vi "Part 2.vi"(11 "Input":string) -> (3 "Output":i64)   [LabVIEW 2021]
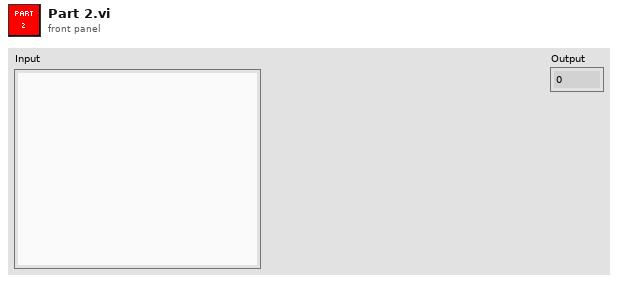
[diagram p1: front panel]
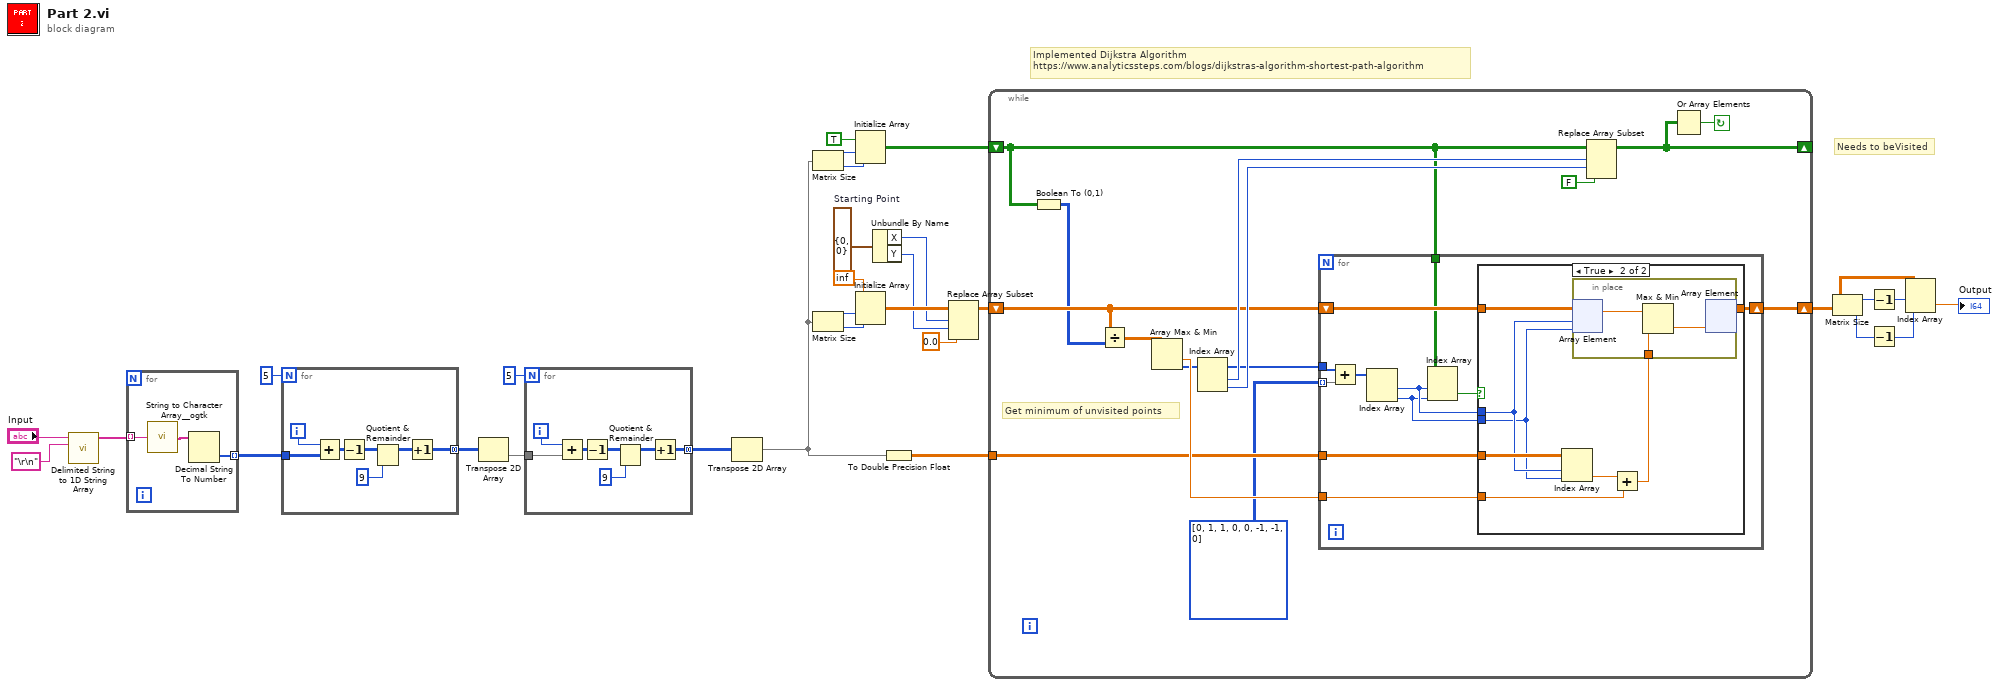
[diagram p0: block diagram]
diagram:
  w18 = cluster{"X":i32, "Y":i32} {"X"=0, "Y"=0}  # Starting Point
  # "Implemented Dijkstra Algorithm\nhttps://www.analyticssteps.com/blogs/dijkstras-algorithm-shortest-path-algorithm"
  # "Needs to beVisited"
  n1 = call <vilib>:"Delimited String to 1D String Array.vi"("delimiter"="\r\n", "delimited string"="Input") -> ("string array"=w29:string[])  [unwired: 9 in]
  n2 = for {
    tunnel: w29 -> [w33] mode=indexing
    tunnel: [w31] -> w9 mode=indexing
    n3 = call <userlib>:"String to Character Array__ogtk.vi"("Input String"=w33) -> ("Character Array"=w32:string[])
    n4 = Decimal String To Number(string=w32) -> (number=w31:i32[])  [unwired: 2 in, 1 out]
  }
  n5 = for {
    N: 5 -> [_]
    tunnel: w9 -> [w39]
    tunnel: [w37] -> w7 mode=concatenating
    i -> [w40]
    n6 = Add(x=w40, y=w39) -> (x+y=w38:i32[][])
    n7 = Decrement(x=w38) -> (x-1=w36:i32[][])
    n8 = Quotient & Remainder(x=w36, y=9) -> (x-y*floor(x/y)=w35:i32[][])  [unwired: 1 out]
    n9 = Increment(x=w35) -> (x+1=w37:i32[][])
  }
  n10 = Transpose 2D Array(2D array=w7) -> (transposed array=w5:i32[][])
  n11 = for {
    N: 5 -> [_]
    tunnel: w5 -> [w46]
    tunnel: [w41] -> w4 mode=concatenating
    i -> [w47]
    n12 = Add(x=w47, y=w46) -> (x+y=w42:i32[][])
    n13 = Decrement(x=w42) -> (x-1=w45:i32[][])
    n14 = Quotient & Remainder(x=w45, y=9) -> (x-y*floor(x/y)=w44:i32[][])  [unwired: 1 out]
    n15 = Increment(x=w44) -> (x+1=w41:i32[][])
  }
  n16 = Transpose 2D Array(2D array=w4) -> (transposed array=w2:i32[][])
  n17 = Matrix Size(0:w2) -> (1:w28:i32, 2:w27:i32)
  n18 = Matrix Size(0:w2) -> (1:w21:i32, 2:w22:i32)
  n19 = Initialize Array(TRUE, w28, w27) -> (w25:bool[][])
  n20 = Initialize Array(inf, w21, w22) -> (w23:dbl[][])
  n21 = Unbundle By Name(w18) -> ("X"=w16:i32, "Y"=w17:i32)
  n22 = To Double Precision Float(number=w2) -> (double precision float=w1:dbl[][])
  n23 = Replace Array Subset(array=w23, new element=0.0, index (row)=w16, index (col)=w17) -> (w19:dbl[][])
  n24 = while {
    shift-right: [w53] -> _
    shift-left: w25 -> [w48]
    shift-right: [w59] -> w10
    shift-left: w19 -> [w55]
    tunnel: w1 -> [w52]
    stop <- w56 continue-if-true
    # "Get minimum of unvisited points"
    n25 = Boolean To (0,1)(Boolean=w48) -> (0, 1=w51:i16[][])
    n26 = Divide(x=w55, y=w51) -> (x/y=w54:dbl[][])
    n27 = Array Max & Min(array=w54) -> (min value=w60:dbl, min index (indices)=w50:i32[])  [unwired: 2 out]
    n28 = Index Array(array=w50) -> (element #1=w58:i32, element #2=w57:i32)  [unwired: 2 in]
    n29 = for {
      tunnel: w60 -> [w72]
      shift-right: [w69] -> w59
      shift-left: w55 -> [w70]
      tunnel: w52 -> [w71]
      tunnel: w50 -> [w67]
      tunnel: i32[][] [[0, 1], [1, 0], [0, -1], [-1, 0]] -> [w68] mode=indexing
      tunnel: w48 -> [w65]
      n30 = Add(x=w67, y=w68) -> (x+y=w66:i32[])
      n31 = Index Array(array=w66) -> (element #1=w63:i32, element #2=w62:i32)  [unwired: 2 in]
      n32 = Index Array(array=w65, index (row)=w63, index (col)=w62) -> (element=w64:bool)
      n33 = case shown="True" w64 {
        tunnel: w72 -> [_ w81]
        tunnel: w71 -> [_ w79]
        tunnel: w70 -> [w73 w78]
        tunnel: [w73 w77] -> w69
        tunnel: w63 -> [_ w76]
        tunnel: w62 -> [_ w75]
        frame False {
        }
        frame True {
          n34 = Index Array(array=w79, index (row)=w76, index (col)=w75) -> (element=w80:dbl)
          n35 = Add(x=w80, y=w81) -> (x+y=w74:dbl)
          n36 = in-place {
            in-place-border: w74 -> [w84]
            n37 = in-place-array #1(w78, w76, w75) -> (w82:dbl)
            n38 = Max & Min(x=w82, y=w84) -> (min(x,y)=w83:dbl)  [unwired: 1 out]
            n39 = in-place-array #1(w83) -> (w77:dbl[][])  [unwired: 2 out]
          }
        }
      }
    }
    n40 = Replace Array Subset(array=w48, new element=FALSE, index (row)=w58, index (col)=w57) -> (w53:bool[][])
    n41 = Or Array Elements(Boolean array=w53) -> (logical OR=w56:bool)
  }
  n42 = Matrix Size(0:w10) -> (1:w15:i32, 2:w13:i32)
  n43 = Decrement(x=w15) -> (x-1=w14:i32)
  n44 = Decrement(x=w13) -> (x-1=w12:i32)
  n45 = Index Array(array=w10, index (row)=w14, index (col)=w12) -> (element=→"Output":dbl)
